vi "Data Logging_Check Validity.vi"(8 "error in":errorcluster, 10 "Data Frame Format":T2={"Absolute Pressure"=TRUE, "Gauge/Diff. Pressure"=TRUE, "Barometric Pressure"=TRUE, "Temperature"=TRUE, "Volumetric"=TRUE, "Mass"=TRUE, "Setpoint"=TRUE, "Valve Drive"=FALSE, "Totalizer"=TRUE, "Totalizer Timer"=FALSE, "Totalizer Average Flow"=FALSE, "Totalizer Peak Flow"=FALSE, "Gas Selected"=TRUE, "Tot. Timer Format"=0}, 11 "Data Logging Options (If valid)":T1={"Absolute Press."=TRUE, "Gauge/Diff. Press."=TRUE, "Barometric Press."=TRUE, "Temperature"=TRUE, "Volumetric"=TRUE, "Mass Flow"=TRUE, "Setpoint"=TRUE, "Valve Drive"=FALSE, "Totalizer"=TRUE, "Tot. Timer [s]"=FALSE, "Tot. Avg. Flow"=FALSE, "Tot. Peak Flow"=FALSE, "Gas Selected"=TRUE, "Log Data"=FALSE}) -> (0 "error out":errorcluster, 2 "Invalid data selected":bool, 3 "Validated Logging Options":T1={"Absolute Press."=TRUE, "Gauge/Diff. Press."=TRUE, "Barometric Press."=TRUE, "Temperature"=TRUE, "Volumetric"=TRUE, "Mass Flow"=TRUE, "Setpoint"=TRUE, "Valve Drive"=FALSE, "Totalizer"=TRUE, "Tot. Timer [s]"=FALSE, "Tot. Avg. Flow"=FALSE, "Tot. Peak Flow"=FALSE, "Gas Selected"=TRUE, "Log Data"=FALSE})   [LabVIEW 2020]
doc: "Check to see if the selected variables to log are present in the Alicat data frame. If invalid data logging options are present, this sub-VI will indicate this with a boolean output, while also outputting the data logging options that are valid with the given Alicat data frame variables."
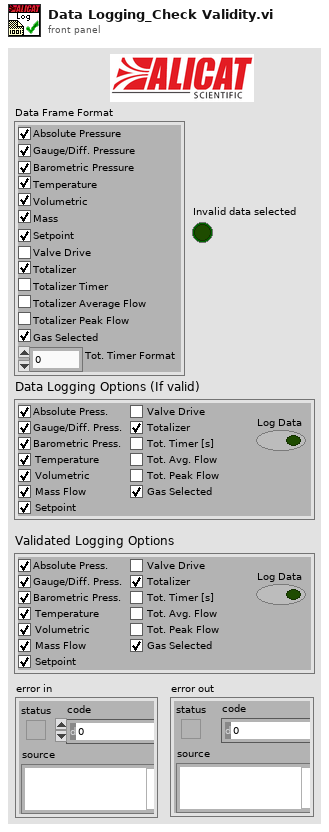
[diagram p1: front panel]
types:
  T1 = cluster{"Absolute Press.":bool, "Gauge/Diff. Press.":bool, "Barometric Press.":bool, "Temperature":bool, "Volumetric":bool, "Mass Flow":bool, "Setpoint":bool, "Valve Drive":bool, "Totalizer":bool, "Tot. Timer [s]":bool, "Tot. Avg. Flow":bool, "Tot. Peak Flow":bool, "Gas Selected":bool, "Log Data":bool}
  T2 = cluster{"Absolute Pressure":bool, "Gauge/Diff. Pressure":bool, "Barometric Pressure":bool, "Temperature":bool, "Volumetric":bool, "Mass":bool, "Setpoint":bool, "Valve Drive":bool, "Totalizer":bool, "Totalizer Timer":bool, "Totalizer Average Flow":bool, "Totalizer Peak Flow":bool, "Gas Selected":bool, "Tot. Timer Format":u16}
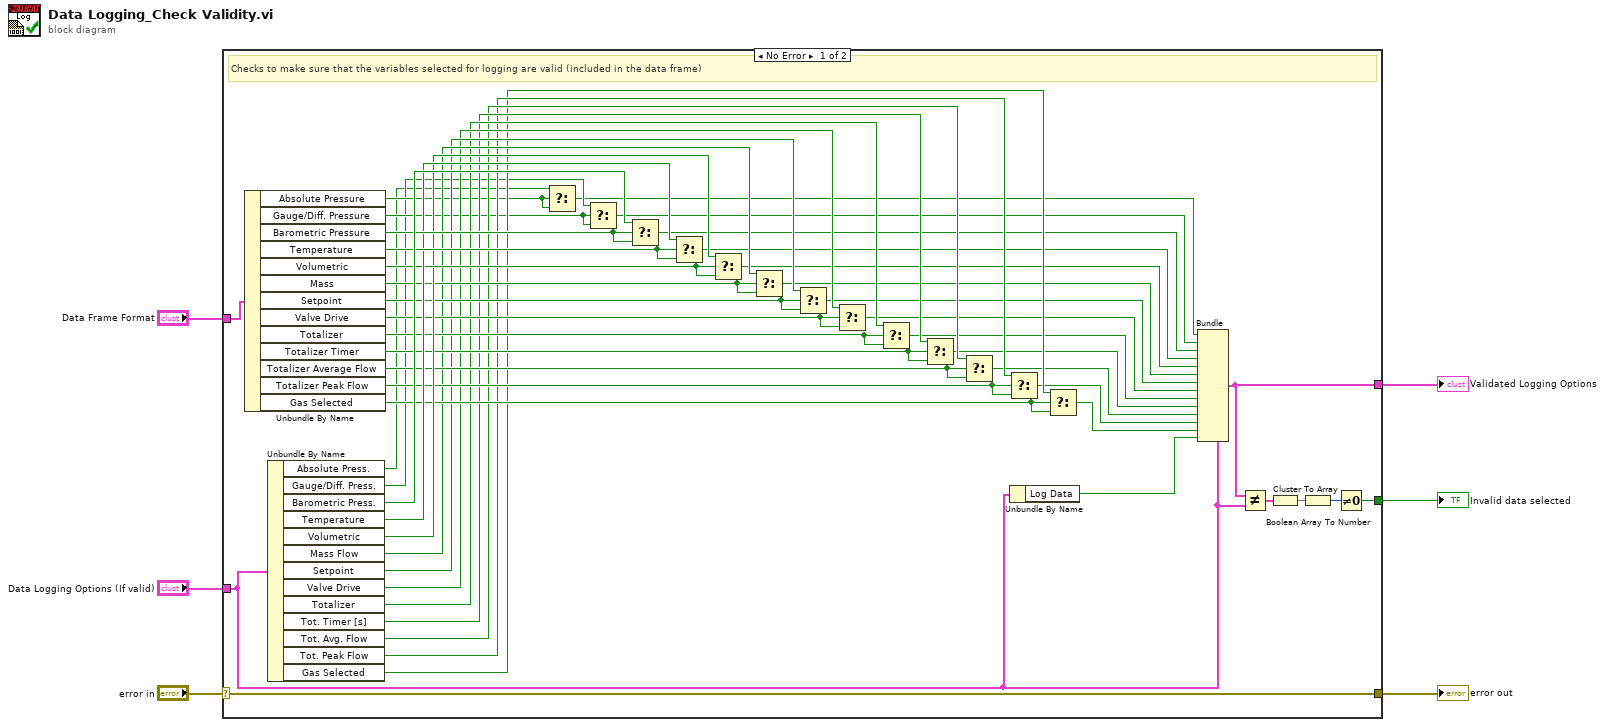
[diagram p0: block diagram]
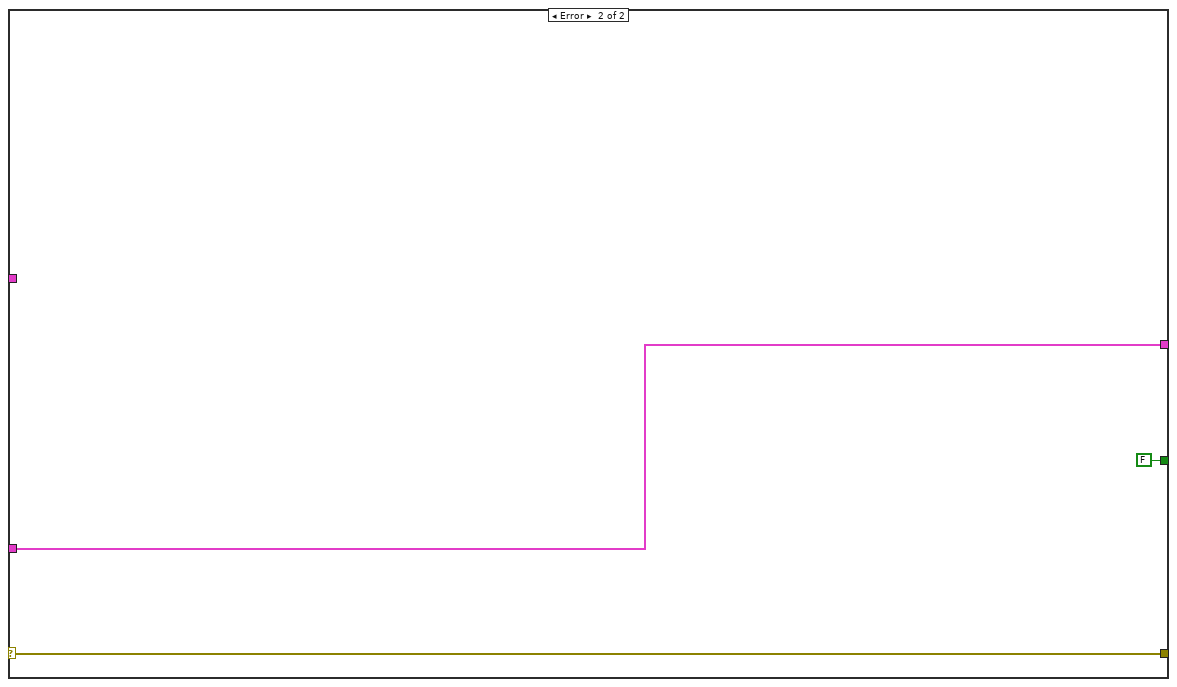
[diagram p2: hidden frame]
diagram:
  n1 = case shown="No Error" "error in" {
    selector: "error in" -> [w54 w57]
    tunnel: "Data Logging Options (If valid)" -> [w30 w55]
    tunnel: [w54 w57] -> w4
    tunnel: "Data Frame Format" -> [w53 _]
    tunnel: [w26 FALSE] -> w2
    tunnel: [w25 w55] -> w1
    frame No Error {
      # "Checks to make sure that the variables selected for logging are valid (included in the data frame)"
      n2 = Unbundle By Name(w53) -> ("Absolute Pressure"=w23:bool, "Gauge/Diff. Pressure"=w24:bool, "Barometric Pressure"=w51:bool, "Temperature"=w50:bool, "Volumetric"=w48:bool, "Mass"=w46:bool, "Setpoint"=w45:bool, "Valve Drive"=w44:bool, "Totalizer"=w43:bool, "Totalizer Timer"=w42:bool, "Totalizer Average Flow"=w41:bool, "Totalizer Peak Flow"=w40:bool, "Gas Selected"=w39:bool)
      n3 = Unbundle By Name(w30) -> ("Absolute Press."=w21:bool, "Gauge/Diff. Press."=w22:bool, "Barometric Press."=w52:bool, "Temperature"=w49:bool, "Volumetric"=w47:bool, "Mass Flow"=w38:bool, "Setpoint"=w37:bool, "Valve Drive"=w36:bool, "Totalizer"=w35:bool, "Tot. Timer [s]"=w34:bool, "Tot. Avg. Flow"=w33:bool, "Tot. Peak Flow"=w32:bool, "Gas Selected"=w31:bool)
      n4 = Select(t=w21, s=w23, f=w23) -> (s? t:f=w7:bool)
      n5 = Select(t=w22, s=w24, f=w24) -> (s? t:f=w8:bool)
      n6 = Select(t=w52, s=w51, f=w51) -> (s? t:f=w9:bool)
      n7 = Select(t=w49, s=w50, f=w50) -> (s? t:f=w10:bool)
      n8 = Select(t=w47, s=w48, f=w48) -> (s? t:f=w11:bool)
      n9 = Select(t=w38, s=w46, f=w46) -> (s? t:f=w12:bool)
      n10 = Select(t=w37, s=w45, f=w45) -> (s? t:f=w13:bool)
      n11 = Select(t=w36, s=w44, f=w44) -> (s? t:f=w14:bool)
      n12 = Select(t=w35, s=w43, f=w43) -> (s? t:f=w15:bool)
      n13 = Select(t=w34, s=w42, f=w42) -> (s? t:f=w16:bool)
      n14 = Select(t=w33, s=w41, f=w41) -> (s? t:f=w17:bool)
      n15 = Select(t=w32, s=w40, f=w40) -> (s? t:f=w18:bool)
      n16 = Unbundle By Name(w30) -> ("Log Data"=w20:bool)
      n17 = Select(t=w31, s=w39, f=w39) -> (s? t:f=w19:bool)
      n18 = Bundle(cluster=w30, "Absolute Press."=w7, "Gauge/Diff. Press."=w8, "Barometric Press."=w9, "Temperature"=w10, "Volumetric"=w11, "Mass Flow"=w12, "Setpoint"=w13, "Valve Drive"=w14, "Totalizer"=w15, "Tot. Timer [s]"=w16, "Tot. Avg. Flow"=w17, "Tot. Peak Flow"=w18, "Gas Selected"=w19, "Log Data"=w20) -> (w25:T1)
      n19 = Not Equal?(x=w25, y=w30) -> (x != y?=w29:T1)
      n20 = Cluster To Array(cluster=w29) -> (array=w28:bool[])
      n21 = Boolean Array To Number(Boolean array=w28) -> (number=w27:u32)
      n22 = Not Equal To 0?(x=w27) -> (x != 0?=w26:bool)
    }
    frame Error {
    }
  }
  "error out" <- w4
  "Invalid data selected" <- w2
  "Validated Logging Options" <- w1
